vi "2_AdvancedDemo_MHHisto.vi"() -> ()   [LabVIEW 2017]
uses:
  Types/MH_InputChannel.ctl
  Types/MH_UIThread_Cmds.ctl
  Types/MH_UIThread_Data.ctl
  _lib/PQ/MultiHarp/MH_InitInfo.ctl
  _lib/PQ/MultiHarp/MH_RefSource.ctl
  _lib/PQ/MultiHarp/MH_MeasMode.ctl
  <vilib>/Utility/error.llb/DialogType.ctl
  _lib/PQ/MultiHarp/mhlib_x86_x64_UIThread.llb/MH_DllPath_global.vi
  <vilib>/Utility/error.llb/Error Cluster From Error Code.vi
  _lib/PQ/MultiHarp/MH_LibVersion_global.vi
  <vilib>/ErrorRing/Error Ring.xnode
panel:
  in  "Settings":bool=TRUE
  in  "Run continuously":bool=TRUE caption="Conti."
  in  "Start":bool
  in  "Scale":bool
  out "CountRates":i32[](graph)
  in  "HistoLength":i32(ring)=6 caption="Num Bins" items=["1024", "2048", "4096", "8192", "16384", "32768", "65536"]
  in  "OvlLevel":u32=100000 caption="Ovl.Level" min=1 step=1
  in  "StopOvl.":bool=TRUE
  in  "AcqTime":i32=1000 caption="Acqu.     ms" min=1 max=360000 step=1
  in  "Binning":i32(ring) caption="Resol.      ps" items=["80", "160", "320", "640", "1280", "2560", "5120", "10240", "20480", "40960", "81920", "163840", "327680", "655360", "1310720", "2621440", "5242880", "10485760", "20971520", "41943040", "83886080", "167772160", "335544320", "671088640", "1342177280", "2684354560"]
  in  "HistoOffset":i32 caption="Offset      ns" min=0 max=100000000 step=1
  out "HistoGraph":T1(graph)={0.0, "Resolution"=0.08, "Histogram"=[]}
  in  "SyncEdge":i32(ring) caption="Edge" items=["falling", "rising"]
  in  "SyncDivider":i32(ring)=3 caption="Divider" items=["1", "2", "4", "8", "16"]
  in  "SyncOffset":i32 caption="Offset      ps" min=-99999 max=99999 step=1
  in  "SyncLevel":i32=-50 caption="Level      mV" min=-1200 max=1200 step=1
  in  "Channels":T2[](array[typedef])=[{"Name"="Inp.Chan 1", "Enable"=TRUE, "Offset"=0, "Level"=-50, "Edge"=0}, {"Name"="Inp.Chan 2", "Enable"=TRUE, "Offset"=0, "Level"=-50, "Edge"=0}, {"Name"="Inp.Chan 3", "Enable"=TRUE, "Offset"=0, "Level"=-50, "Edge"=0}, {"Name"="Inp.Chan 4", "Enable"=TRUE, "Offset"=0, "Level"=-50, "Edge"=0}, {"Name"="Inp.Chan 5", "Enable"=TRUE, "Offset"=0, "Level"=-50, "Edge"=0}, {"Name"="Inp.Chan 6", "Enable"=TRUE, "Offset"=0, "Level"=-50, "Edge"=0}, {"Name"="Inp.Chan 7", "Enable"=TRUE, "Offset"=0, "Level"=-50, "Edge"=0}, {"Name"="Inp.Chan 8", "Enable"=TRUE, "Offset"=0, "Level"=-50, "Edge"=0}] {"Edge" items=["falling", "rising"]; "Offset" min=-99999 max=99999 step=80; "Level" min=-1200 max=1200 step=1}
  out "SyncRate":string="Sync Rate: 10000160 cps\n"
  out "OverFlow":bool caption="Overflow:"
  out "Status":string="Readout Rate: 7.4 Hz\t\tTotal Counts:\t\tCh. 1: 3766 cnts.\t\tCh. 2: 3766 cnts.\t\tCh. 3: 0 cnts.\t\tCh. 4: 0 cnts.\t\tCh. 5: 0 cnts.\t\tCh. 6: 0 cnts.\t\tCh. 7: 0 cnts.\t\tCh. 8: 0 cnts.\t\t"
  # "Histogram"
  # "Sync"
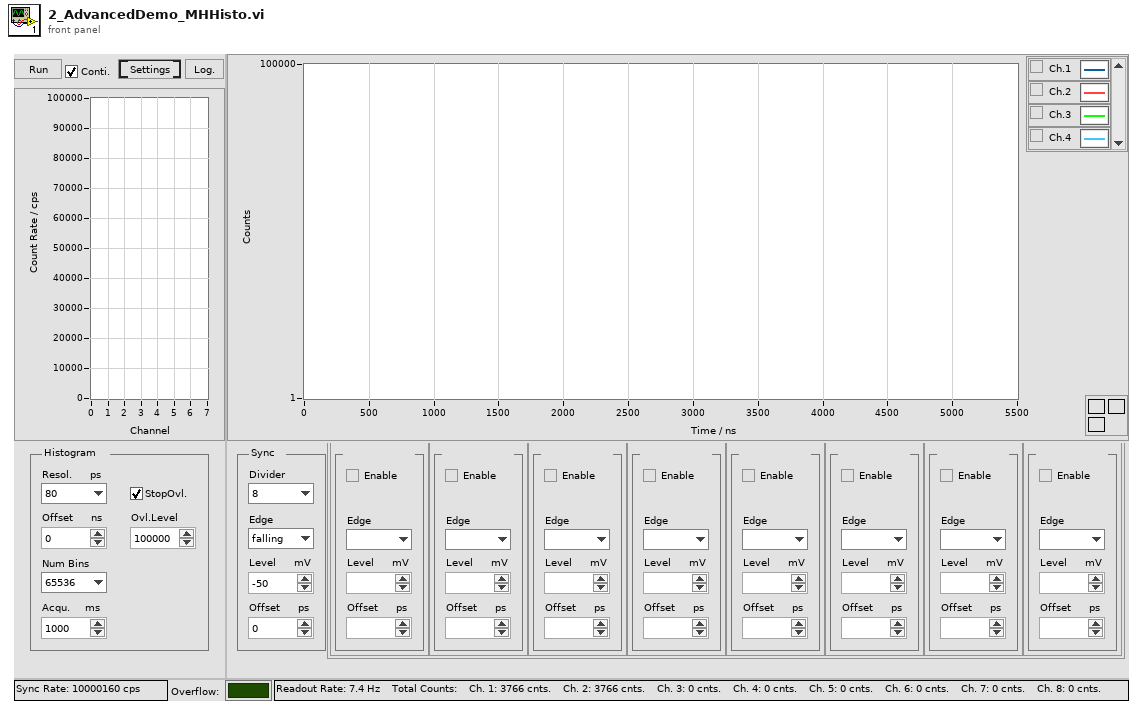
[diagram p1: front panel]
types:
  T1 = cluster{dbl, "Resolution":dbl, "Histogram":u32[][]}
  T2 = typedef "MH_InputChannel.ctl" = cluster{"Name":string, "Enable":bool, "Offset":i32, "Level":i32, "Edge":i32}
  T3 = typedef "MH_UIThread_Data.ctl" = cluster{"Init Info":T4, "DevIdx":i32, "SyncDivider":i32, "SyncOffset":i32, "SyncLevel":i32, "Channels":T2[], "CurrentChannels":i32[], "AcqTime":i32, "Binning":i32, "HistoOffset":i32, "HistoLen":i32, "StopOvl.":bool, "OvlLevel":u32, "SyncEdge":i32, "StartMeas":bool, "HistoLength":i32, "Resolution":dbl, "Run cont.":bool, "Status":string, "SyncRate":i32, "BitShift":i32, "HistoAcqTime":dbl}
  T4 = typedef "MH_InitInfo.ctl" = cluster{"Library Version":string, "Serial No.":string, "Model":string, "Partnum":string, "Version":string, "features":i32, "nchannels":i32, "Base Resolution":dbl, "Bin Steps":i32}
  T5 = typedef "MH_UIThread_Cmds.ctl" = enum16{"Idle", "Init", "SetInpChanEnable", "SetInpChanOffset", "SetInpChanTrg", "SetSyncDivider", "SetSyncTrg", "SetSyncOffset", "SetBinning", "SetHistoOffset", "SetHistoLen", "SetStopOvl", "SetBitShift", "SetHistoAcqTime", "GetRates", "GetAllRates", "StartMeas", "StopMeas", "AbortMeas", "GetResolution", "GetHistos", "GetAllHistos", "ReadFiFo", "WriteStatus", "Resize", "EnableControls", "DisableControls", "Error", "Exit"}
  T6 = enum8{"Enabled", "Disabled", "Disabled and Grayed Out"}
  T7 = typedef "MH_MeasMode.ctl" = i32
  T8 = typedef "MH_RefSource.ctl" = enum16{"INTERNAL", "EXTERNAL_10MHZ", "WR_MASTER_GENERIC", "WR_SLAVE_GENERIC", "WR_GRANDM_GENERIC", "EXTN_GPS_PPS", "EXTN_GPS_PPS_UART", "WR_MASTER_MHARP", "WR_SLAVE_MHARP", "WR_GRANDM_MHARP"}
  T9 = cluster{dbl, "Resolution":dbl, "Histograms":u32[][]}
  T10 = typedef "DialogType.ctl" = u16
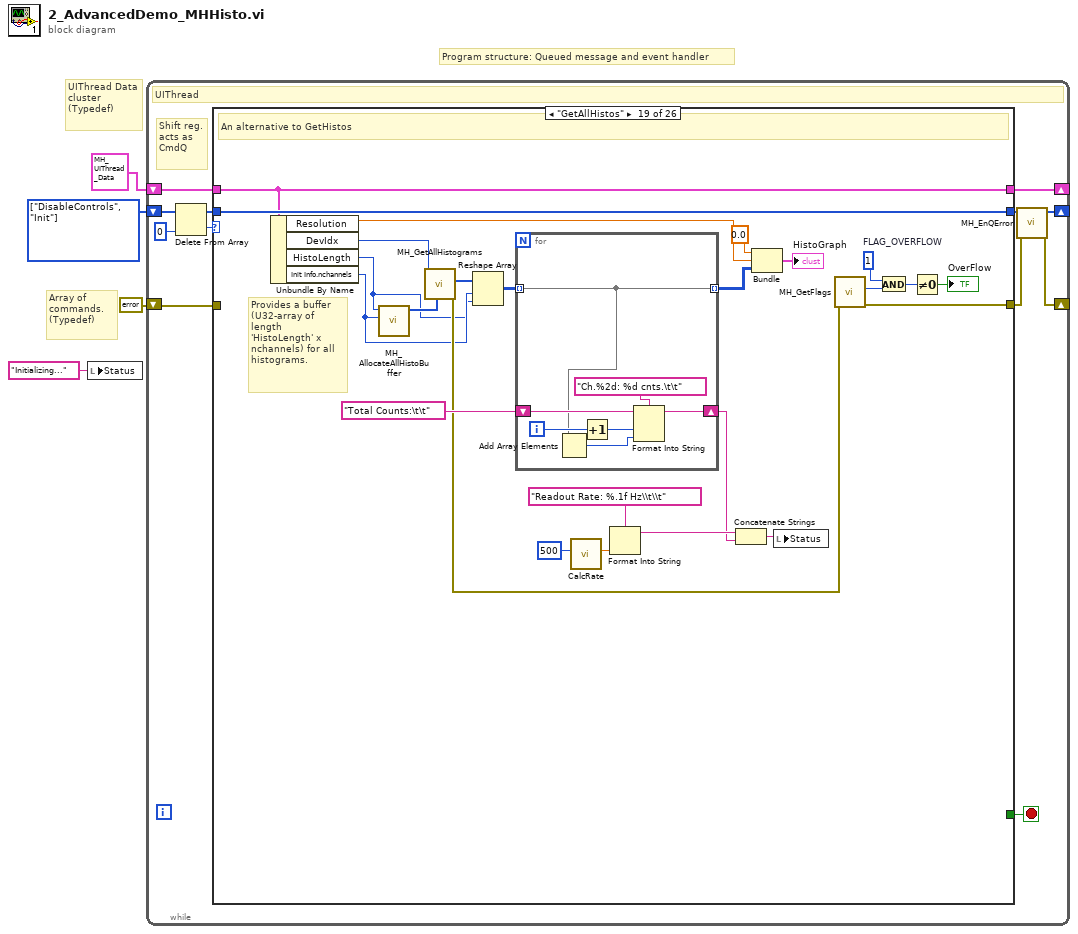
[diagram p0: block diagram]
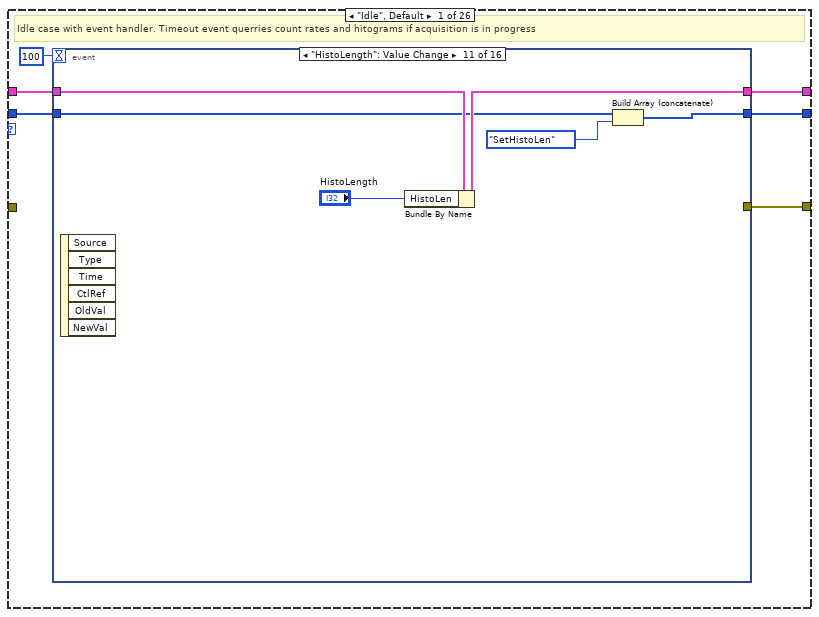
[diagram p2: hidden frame]
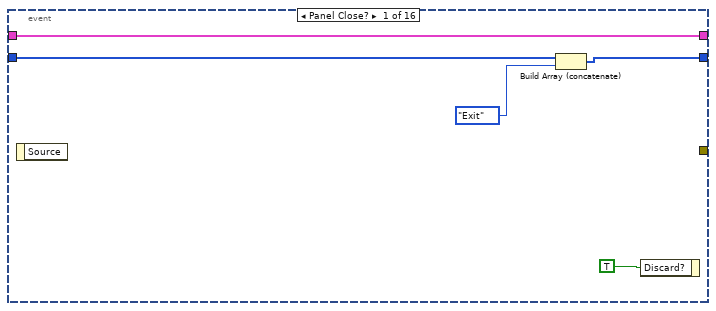
[diagram p3: hidden frame]
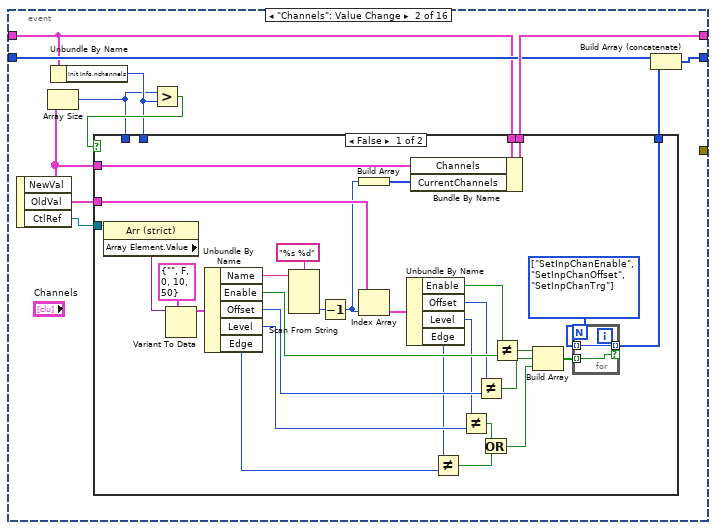
[diagram p4: hidden frame]
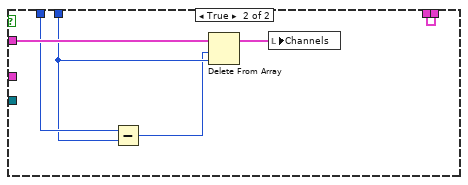
[diagram p5: hidden frame]
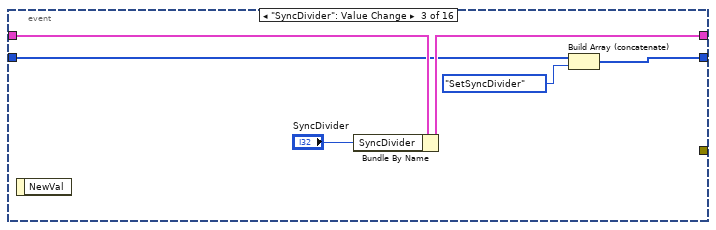
[diagram p6: hidden frame]
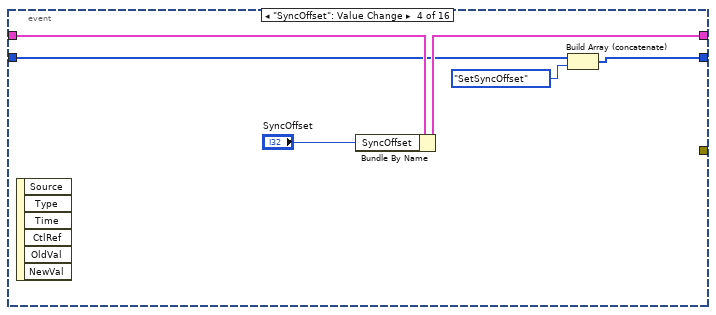
[diagram p7: hidden frame]
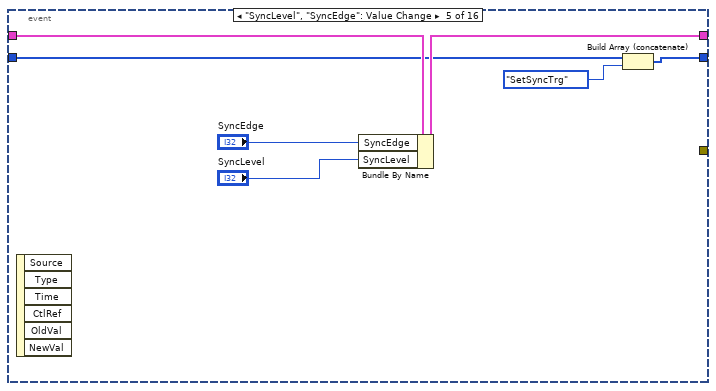
[diagram p8: hidden frame]
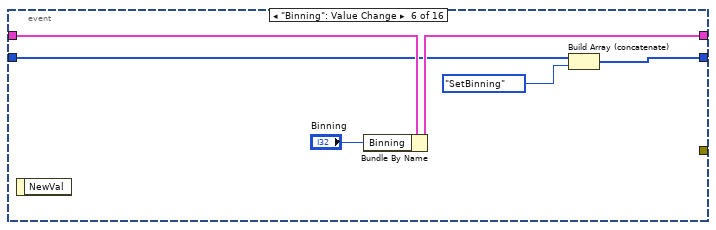
[diagram p9: hidden frame]
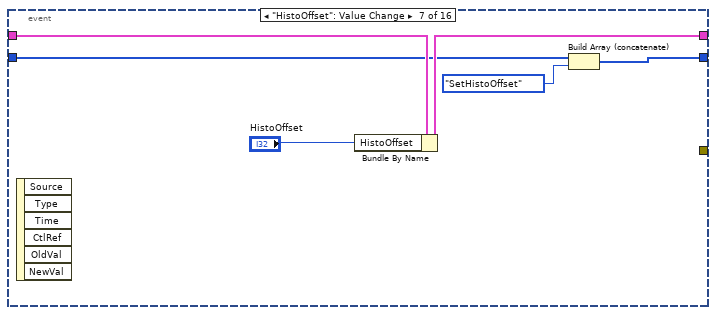
[diagram p10: hidden frame]
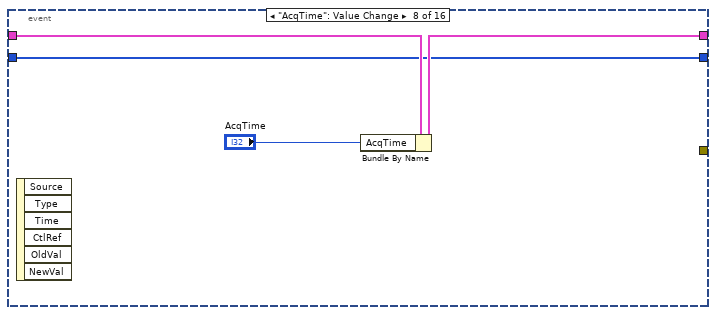
[diagram p11: hidden frame]
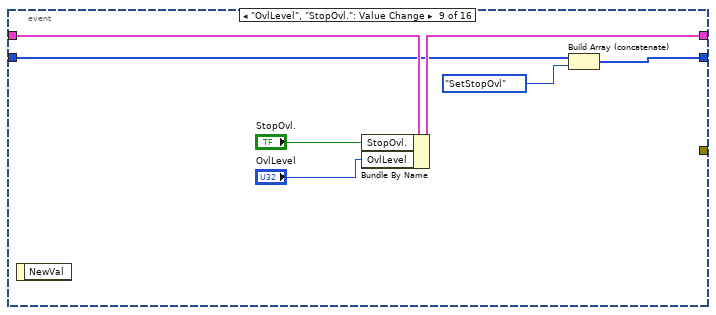
[diagram p12: hidden frame]
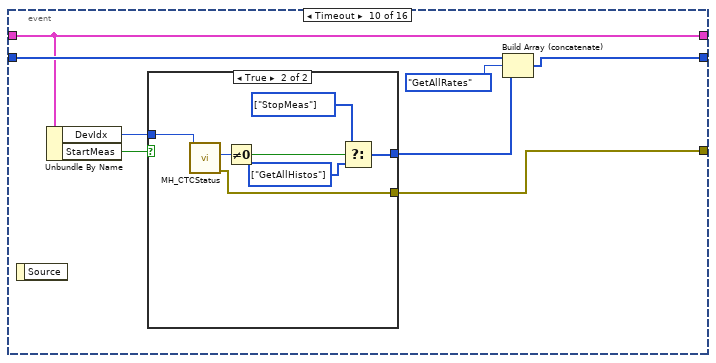
[diagram p13: hidden frame]
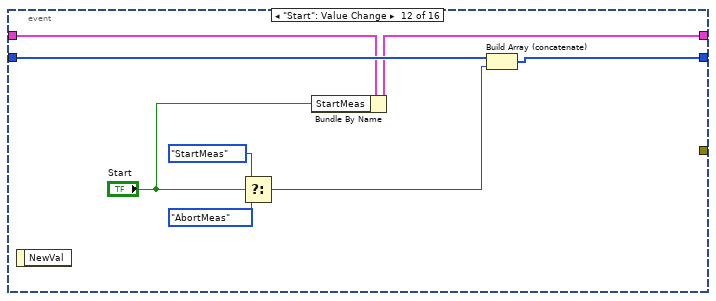
[diagram p15: hidden frame]
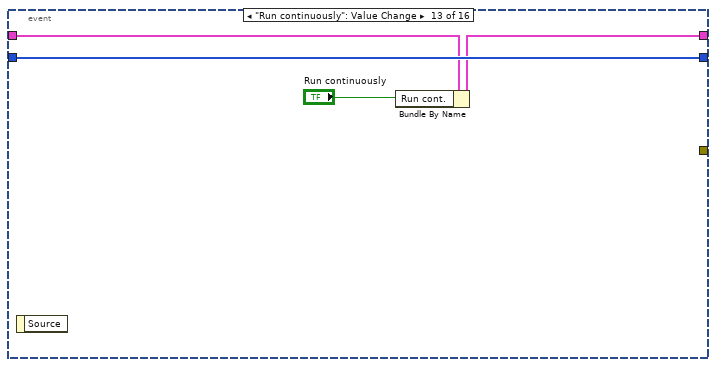
[diagram p16: hidden frame]
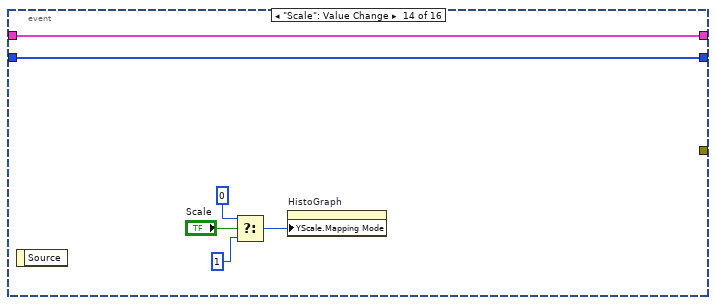
[diagram p17: hidden frame]
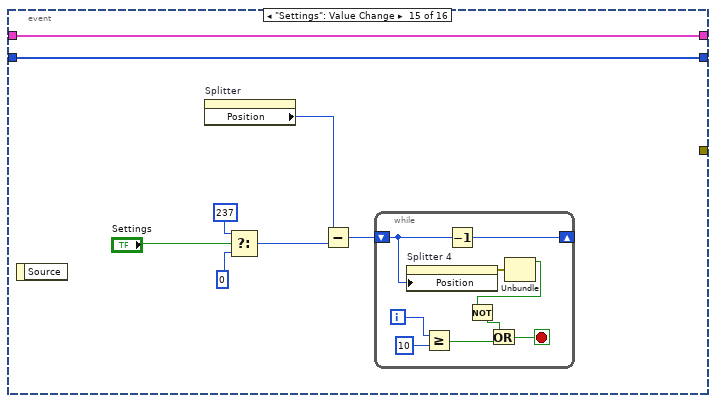
[diagram p18: hidden frame]
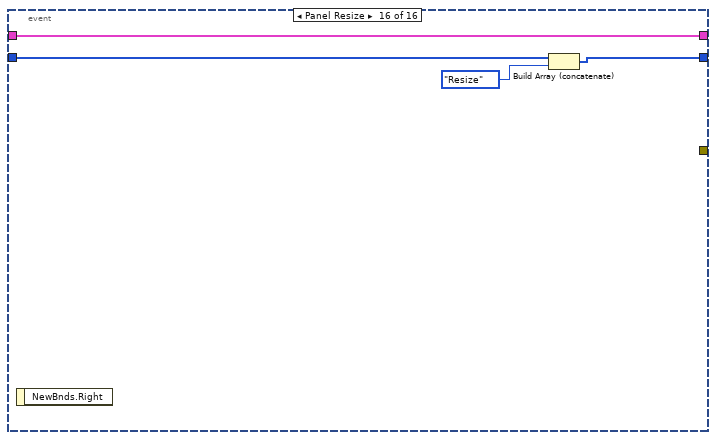
[diagram p19: hidden frame]
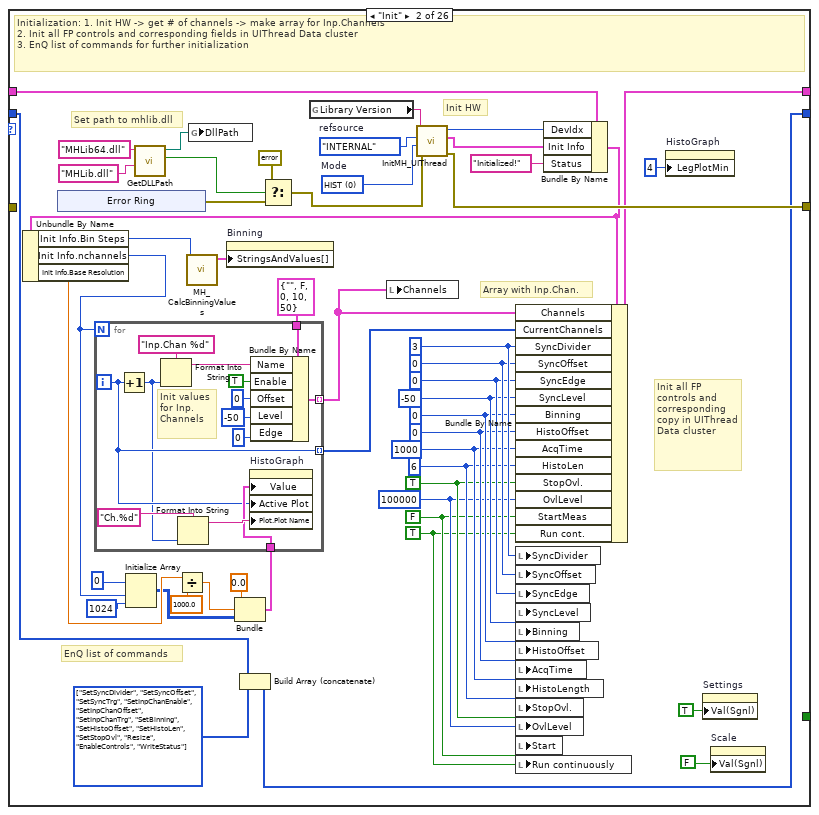
[diagram p20: hidden frame]
diagram:
  w3 = T5[] [enum."DisableControls", enum."Init"] items=["Idle", "Init", "SetInpChanEnable", "SetInpChanOffset", "SetInpChanTrg", "SetSyncDivider", "SetSyncTrg", "SetSyncOffset", "SetBinning", "SetHistoOffset", "SetHistoLen", "SetStopOvl", "SetBitShift", "SetHistoAcqTime", "GetRates", "GetAllRates", "StartMeas", "StopMeas", "AbortMeas", "GetResolution", "GetHistos", "GetAllHistos", "ReadFiFo", "WriteStatus", "Resize", "EnableControls", "DisableControls", "Error", "Exit"]
  # "Array of commands.\n(Typedef)"
  # "Program structure: Queued message and event handler"
  # "UIThread Data cluster\n(Typedef)"
  n1 = local write "Status"("Initializing..." ("Status")) -> ()
  n2 = while {
    shift-right: [w5] -> _
    shift-left: w3 -> [w12]
    shift-right: [w15] -> _
    shift-left: T3 {"Init Info"={"Library Version"="", "Serial No."="", "Model"="", "Partnum"="", "Version"="", "features"=0, "nchannels"=0, "Base Resolution"=0.0, "Bin Steps"=0}, "DevIdx"=0, "SyncDivider"=1, "SyncOffset"=0, "SyncLevel"=50, "Channels"=[], "CurrentChannels"=[], "AcqTime"=1, "Binning"=1, "HistoOffset"=1, "HistoLen"=1024, "StopOvl."=FALSE, "OvlLevel"=1024, "SyncEdge"=10, "StartMeas"=FALSE, "HistoLength"=0, "Resolution"=0.0, "Run cont."=FALSE, "Status"="", "SyncRate"=0, "BitShift"=0, "HistoAcqTime"=0.0} -> [w14]
    shift-right: [w7] -> _
    shift-left: errorcluster {"status"=FALSE, "code"=0, "source"=""} ("error IO") -> [w13]
    stop <- w16 stop-if-true
    # "Shift reg.\nacts as\nCmdQ"
    # "UIThread"
    n3 = Delete From Array(array=w12, index=0) -> (deleted portion=w10:T5, array with subset deleted=w9:T5[])  [unwired: 1 in]
    n4 = case shown="\"GetAllHistos\"" w10 {
      tunnel: [w22 w221 w249 w263 w277 w294 w303 w305 w312 w320 w328 w333 w344 w355 w370 w378 w392 w406 w431 w463 w487 w500 w507 w519 w525 w529] -> w6
      tunnel: [_ _ _ _ _ _ _ _ _ _ _ _ _ _ _ _ _ _ _ _ _ _ _ _ _ TRUE] -> w16
      tunnel: [w21 w201 w252 w266 w280 w296 w304 w309 w316 w321 w323 w334 w343 w354 w376 w381 w395 w402 w430 w462 w486 w488 w506 w518 w526 w532] -> w15
      tunnel: w14 -> [w20 w206 w252 w266 w280 w296 w304 w309 w316 w321 w324 w334 w343 w354 w376 w382 w396 w403 w430 w462 w486 w488 w506 w518 w526 w532]
      tunnel: [w17 w224 w250 w264 w278 w292 w302 w308 w315 w319 w327 w332 w337 w353 w375 w384 w398 w404 w428 w458 _ _ _ _ _ w530] -> w8
      tunnel: w13 -> [_ _ _ _ _ _ _ _ _ _ _ _ _ _ _ _ _ _ _ _ _ _ _ _ w527 _]
      tunnel: w9 -> [w19 w223 w249 w263 w277 w294 w303 w305 w311 w320 w328 w333 w344 w355 w371 w379 w393 w406 w431 w463 w487 w500 w507 w519 _ w529]
      frame "Idle", Default {
        # "Idle case with event handler. Timeout event querries count rates and hitograms if acquisition is in progress"
        n5 = event shown="[10] \"HistoLength\": Value Change" {
          selector: _ -> [_ _ _ _ _ _ _ _ _ _ _ _ _ _ _ _]
          dyn-events: _ -> [_ _ _ _ _ _ _ _ _ _ _ _ _ _ _ _]
          timeout: 100 -> [_ _ _ _ _ _ _ _ _ _ _ _ _ _ _ _]
          tunnel: [w23 w33 w77 w83 w90 w97 w103 w108 w114 w124 w135 w143 w151 w157 w165 w175] -> w22
          tunnel: [w26 w36 w81 w87 w94 w100 w106 w110 w117 w123 w138 w141 w149 w156 w164 w178] -> w21
          tunnel: w20 -> [w26 w32 w82 w88 w95 w101 w107 w111 w118 w123 w139 w142 w150 w156 w164 w178]
          tunnel: w19 -> [w25 w35 w79 w85 w92 w99 w105 w108 w116 w126 w137 w145 w151 w157 w165 w176]
          tunnel: [_ _ _ _ _ _ _ _ _ w119 _ _ _ _ _ _] -> w17
          event Panel Close? {
            n6 = event-data() -> ()  [unwired: 1 in, 1 out]
            n7 = Build Array (concatenate)(w25, MH_UIThread_Cmds."Exit") -> (w23:T5[])
            n8 = event-data("Discard?"=TRUE) -> ()  [unwired: 1 in, 1 out]
          }
          event "Channels": Value Change {
            n9 = event-data() -> ("NewVal"=w31:T2[], "OldVal"=w37:T2[], "CtlRef"=w38:refnum<vi>)  [unwired: 1 in]
            n10 = Array Size(array=w31) -> (size(s)=w28:i32)
            n11 = Unbundle By Name(w32) -> ("Init Info.nchannels"=w29:i32)
            n12 = Greater?(x=w28, y=w29) -> (0:w30:bool)
            n13 = case shown="False" w30 {
              tunnel: w38 -> [w68 _]
              tunnel: w37 -> [w62 _]
              tunnel: [w45 w76] -> w36
              tunnel: [w43 _] -> w34
              tunnel: w32 -> [w40 w76]
              tunnel: w31 -> [w39 w75]
              tunnel: w29 -> [_ w73]
              tunnel: w28 -> [_ w74]
              frame False {
                w46 = T5[] [enum."SetInpChanEnable", enum."SetInpChanOffset", enum."SetInpChanTrg"] items=["Idle", "Init", "SetInpChanEnable", "SetInpChanOffset", "SetInpChanTrg", "SetSyncDivider", "SetSyncTrg", "SetSyncOffset", "SetBinning", "SetHistoOffset", "SetHistoLen", "SetStopOvl", "SetBitShift", "SetHistoAcqTime", "GetRates", "GetAllRates", "StartMeas", "StopMeas", "AbortMeas", "GetResolution", "GetHistos", "GetAllHistos", "ReadFiFo", "WriteStatus", "Resize", "EnableControls", "DisableControls", "Error", "Exit"]
                n14 = property class="Arr (strict)"(reference=w68) -> ("Array Element.Value"=w67:variant)  [unwired: 1 in, 2 out]
                n15 = Variant To Data(type=T2 {"Name"="", "Enable"=FALSE, "Offset"=0, "Level"=10, "Edge"=50} ("Channel"), Variant=w67) -> (data=w44:T2)  [unwired: 1 in, 1 out]
                n16 = Unbundle By Name(w44) -> ("Name"=w65:string, "Enable"=w59:bool, "Offset"=w57:i32, "Level"=w55:i32, "Edge"=w53:i32)
                n17 = Scan From String(format string="%s %d", input string=w65) -> (output 2=w63:i32)  [unwired: 5 in, 3 out]
                n18 = Decrement(x=w63) -> (x-1=w42:i32)
                n19 = Build Array(w42) -> (w41:i32[])
                n20 = Index Array(array=w62, index=w42) -> (element=w61:T2)
                n21 = Unbundle By Name(w61) -> ("Enable"=w60:bool, "Offset"=w58:i32, "Level"=w56:i32, "Edge"=w54:i32)
                n22 = Bundle By Name(cluster=w40, "Channels"=w39, "CurrentChannels"=w41) -> (w45:T3)
                n23 = Not Equal?(x=w54, y=w53) -> (x != y?=w48:bool)
                n24 = Not Equal?(x=w56, y=w55) -> (x != y?=w49:bool)
                n25 = Not Equal?(x=w58, y=w57) -> (x != y?=w51:bool)
                n26 = Or(x=w49, y=w48) -> (x .or. y?=w47:bool)
                n27 = Not Equal?(x=w60, y=w59) -> (x != y?=w52:bool)
                n28 = Build Array(w52, w51, w47) -> (w50:bool[])
                n29 = for {
                  tunnel: w50 -> [w69] mode=indexing
                  tunnel: w46 -> [w70] mode=indexing
                  tunnel: [w70] -> w43 mode=indexing if=w69
                }
              }
              frame True {
                n30 = Subtract(x=w74, y=w73) -> (x-y=w72:i32)
                n31 = Delete From Array(array=w75, length=w72, index=w73) -> (array with subset deleted=w71:T2[])  [unwired: 1 out]
                n32 = local write "Channels"(w71) -> ()
              }
            }
            n33 = Build Array (concatenate)(w35, w34) -> (w33:T5[])
          }
          event "SyncDivider": Value Change {
            n34 = event-data() -> ()  [unwired: 1 in, 1 out]
            n35 = Bundle By Name(cluster=w82, "SyncDivider"="SyncDivider") -> (w81:T3)
            n36 = Build Array (concatenate)(w79, MH_UIThread_Cmds."SetSyncDivider") -> (w77:T5[])
          }
          event "SyncOffset": Value Change {
            n37 = event-data() -> ()  [unwired: 1 in, 6 out]
            n38 = Bundle By Name(cluster=w88, "SyncOffset"="SyncOffset") -> (w87:T3)
            n39 = Build Array (concatenate)(w85, MH_UIThread_Cmds."SetSyncOffset") -> (w83:T5[])
          }
          event "SyncLevel", "SyncEdge": Value Change {
            n40 = event-data() -> ()  [unwired: 1 in, 6 out]
            n41 = Bundle By Name(cluster=w95, "SyncEdge"="SyncEdge", "SyncLevel"="SyncLevel") -> (w94:T3)
            n42 = Build Array (concatenate)(w92, MH_UIThread_Cmds."SetSyncTrg") -> (w90:T5[])
          }
          event "Binning": Value Change {
            n43 = event-data() -> ()  [unwired: 1 in, 1 out]
            n44 = Bundle By Name(cluster=w101, "Binning"="Binning") -> (w100:T3)
            n45 = Build Array (concatenate)(w99, MH_UIThread_Cmds."SetBinning") -> (w97:T5[])
          }
          event "HistoOffset": Value Change {
            n46 = event-data() -> ()  [unwired: 1 in, 6 out]
            n47 = Bundle By Name(cluster=w107, "HistoOffset"="HistoOffset") -> (w106:T3)
            n48 = Build Array (concatenate)(w105, MH_UIThread_Cmds."SetHistoOffset") -> (w103:T5[])
          }
          event "AcqTime": Value Change {
            n49 = event-data() -> ()  [unwired: 1 in, 6 out]
            n50 = Bundle By Name(cluster=w111, "AcqTime"="AcqTime") -> (w110:T3)
          }
          event "OvlLevel", "StopOvl.": Value Change {
            n51 = event-data() -> ()  [unwired: 1 in, 1 out]
            n52 = Bundle By Name(cluster=w118, "StopOvl."="StopOvl.", "OvlLevel"="OvlLevel") -> (w117:T3)
            n53 = Build Array (concatenate)(w116, MH_UIThread_Cmds."SetStopOvl") -> (w114:T5[])
          }
          event Timeout {
            n54 = event-data() -> ()  [unwired: 1 in, 1 out]
            n55 = Unbundle By Name(w123) -> ("DevIdx"=w121:i32, "StartMeas"=w122:bool)
            n56 = case shown="True" w122 {
              tunnel: w121 -> [_ w133]
              tunnel: [_ w131] -> w120
              tunnel: [_ w128] -> w119
              frame False {
              }
              frame True {
                w129 = T5[] [enum."GetAllHistos"] items=["Idle", "Init", "SetInpChanEnable", "SetInpChanOffset", "SetInpChanTrg", "SetSyncDivider", "SetSyncTrg", "SetSyncOffset", "SetBinning", "SetHistoOffset", "SetHistoLen", "SetStopOvl", "SetBitShift", "SetHistoAcqTime", "GetRates", "GetAllRates", "StartMeas", "StopMeas", "AbortMeas", "GetResolution", "GetHistos", "GetAllHistos", "ReadFiFo", "WriteStatus", "Resize", "EnableControls", "DisableControls", "Error", "Exit"]
                w130 = T5[] [enum."StopMeas"] items=["Idle", "Init", "SetInpChanEnable", "SetInpChanOffset", "SetInpChanTrg", "SetSyncDivider", "SetSyncTrg", "SetSyncOffset", "SetBinning", "SetHistoOffset", "SetHistoLen", "SetStopOvl", "SetBitShift", "SetHistoAcqTime", "GetRates", "GetAllRates", "StartMeas", "StopMeas", "AbortMeas", "GetResolution", "GetHistos", "GetAllHistos", "ReadFiFo", "WriteStatus", "Resize", "EnableControls", "DisableControls", "Error", "Exit"]
                n57 = call "MH_CTCStatus.vi"("devidx"=w133) -> ("error out"=w128:errorcluster, "ctcstatus"=w132:i32)  [unwired: 8 in, 1 out]
                n58 = Not Equal To 0?(x=w132) -> (x != 0?=w127:bool)
                n59 = Select(t=w130, s=w127, f=w129) -> (s? t:f=w131:T5[])
              }
            }
            n60 = Build Array (concatenate)(w126, MH_UIThread_Cmds."GetAllRates", w120) -> (w124:T5[])
          }
          event "HistoLength": Value Change {
            n61 = event-data() -> ()  [unwired: 1 in, 6 out]
            n62 = Bundle By Name(cluster=w139, "HistoLen"="HistoLength") -> (w138:T3)
            n63 = Build Array (concatenate)(w137, MH_UIThread_Cmds."SetHistoLen") -> (w135:T5[])
          }
          event "Start": Value Change {
            n64 = event-data() -> ()  [unwired: 1 in, 1 out]
            n65 = Select(t=MH_UIThread_Cmds."StartMeas", s="Start", f=MH_UIThread_Cmds."AbortMeas") -> (s? t:f=w144:T5)
            n66 = Bundle By Name(cluster=w142, "StartMeas"="Start") -> (w141:T3)
            n67 = Build Array (concatenate)(w145, w144) -> (w143:T5[])
          }
          event "Run continuously": Value Change {
            n68 = event-data() -> ()  [unwired: 1 in, 1 out]
            n69 = Bundle By Name(cluster=w150, "Run cont."="Run continuously") -> (w149:T3)
          }
          event "Scale": Value Change {
            n70 = event-data() -> ()  [unwired: 1 in, 1 out]
            n71 = Select(t=u8 0 ("Y Scale.Mapping Mode"), s="Scale", f=u8 1 ("Y Scale.Mapping Mode")) -> (s? t:f=w152:u8)
            n72 = property on="HistoGraph" class="WFGraph (strict)"("YScale.Mapping Mode"=w152) -> ()  [unwired: 2 in, 2 out]
          }
          event "Settings": Value Change {
            n73 = event-data() -> ()  [unwired: 1 in, 1 out]
            n74 = property on="Splitter" class="Splitter"() -> ("Position"=w163:i32)  [unwired: 2 in, 2 out]
            n75 = Select(t=237 ("PosT"), s="Settings", f=0 ("PosF")) -> (s? t:f=w160:i32)
            n76 = Subtract(x=w163, y=w160) -> (x-y=w159:i32)
            n77 = while {
              shift-right: [w174] -> _
              shift-left: w159 -> [w167]
              i -> [w173]
              stop <- w170 stop-if-true
              n78 = property on="Splitter 4" class="Splitter"("Position"=w167) -> (error out=w166:errorcluster)  [unwired: 2 in, 1 out]
              n79 = Greater Or Equal?(x=w173, y=10) -> (x >= y?=w171:bool)
              n80 = Decrement(x=w167) -> (x-1=w174:i32)
              n81 = Unbundle(w166) -> ("status"=w169:bool)  [unwired: 2 out]
              n82 = Not(x=w169) -> (.not. x?=w168:bool)
              n83 = Or(x=w168, y=w171) -> (x .or. y?=w170:bool)
            }
          }
          event Panel Resize {
            n84 = event-data() -> ()  [unwired: 1 in, 1 out]
            n85 = Build Array (concatenate)(w176, MH_UIThread_Cmds."Resize") -> (w175:T5[])
          }
        }
      }
      frame "Init" {
        w179 = T7 0 items=["HIST"=0, "T2"=2, "T3"=3]  # Mode
        w193 = MH_RefSource."INTERNAL"  # refsource
        w208 = TRUE ("Run cont.")
        w210 = FALSE ("StartMeas")
        w211 = u32 100000 ("OvlLevel")
        w212 = TRUE ("StopOvl.")
        w213 = 6 ("HistoLen")
        w214 = 1000 ("AcqTime")
        w215 = 0 ("HistoOffset")
        w216 = 0 ("Binning")
        w217 = -50 ("SyncLevel")
        w218 = 0 ("SyncZeroX")
        w219 = 0 ("SyncOffset")
        w220 = 3 ("SyncDivider")
        w222 = T5[] [enum."SetSyncDivider", enum."SetSyncOffset", enum."SetSyncTrg", enum."SetInpChanEnable", enum."SetInpChanOffset", enum."SetInpChanTrg", enum."SetBinning", enum."SetHistoOffset", enum."SetHistoLen", enum."SetStopOvl", enum."Resize", enum."EnableControls", enum."WriteStatus"] items=["Idle", "Init", "SetInpChanEnable", "SetInpChanOffset", "SetInpChanTrg", "SetSyncDivider", "SetSyncTrg", "SetSyncOffset", "SetBinning", "SetHistoOffset", "SetHistoLen", "SetStopOvl", "SetBitShift", "SetHistoAcqTime", "GetRates", "GetAllRates", "StartMeas", "StopMeas", "AbortMeas", "GetResolution", "GetHistos", "GetAllHistos", "ReadFiFo", "WriteStatus", "Resize", "EnableControls", "DisableControls", "Error", "Exit"]
        # "Init HW"
        # "Set path to mhlib.dll"
        # "Init all FP controls and corresponding copy in UIThread Data cluster"
        # "EnQ list of commands"
        # "Array with Inp.Chan."
        # "Initialization: 1. Init HW -> get # of channels -> make array for Inp.Channels\n2. Init all FP controls and corresponding fields in UIThread Data cluster\n3. EnQ list of commands for further initialization"
        n86 = xnode "Error Ring"() -> ("error out"=w194:errorcluster)
        n87 = call "GetDLLPath.vi"("DllName_32bit"="MHLib.dll" ("name or relative path"), "DllName_64bit"="MHLib64.dll" ("name or relative path")) -> ("file exists?"=w196:bool, "DLLPath"=w197:path)  [unwired: 8 in]
        n88 = global write "MH_DllPath_global.vi" "DllPath"(w197) -> ()
        n89 = Build Array (concatenate)(w223, w222) -> (w221:T5[])
        n90 = Select(t=errorcluster {"status"=FALSE, "code"=0, "source"=""} ("error IO"), s=w196, f=w194) -> (s? t:f=w202:errorcluster)
        n91 = global read "MH_LibVersion_global.vi" "Library Version"() -> (w192:string)
        n92 = call "InitMH_UIThread.vi"("error in (no error)"=w202, "Mode"=w179, "refsource"=w193, "Library Version"=w192) -> ("error out"=w224:errorcluster, "Init Info"=w227:T4, "DevIdx"=w226:i32)  [unwired: 5 in]
        n93 = local write "SyncDivider"(w220) -> ()
        n94 = local write "SyncOffset"(w219) -> ()
        n95 = local write "SyncEdge"(w218) -> ()
        n96 = local write "SyncLevel"(w217) -> ()
        n97 = local write "Binning"(w216) -> ()
        n98 = local write "HistoOffset"(w215) -> ()
        n99 = local write "AcqTime"(w214) -> ()
        n100 = local write "HistoLength"(w213) -> ()
        n101 = local write "StopOvl."(w212) -> ()
        n102 = local write "OvlLevel"(w211) -> ()
        n103 = local write "Start"(w210) -> ()
        n104 = local write "Run continuously"(w208) -> ()
        n105 = Bundle By Name(cluster=w206, "DevIdx"=w226, "Init Info"=w227, "Status"="Initialized!") -> (w205:T3)
        n106 = Unbundle By Name(w205) -> ("Init Info.Bin Steps"=w204:i32, "Init Info.nchannels"=w181:i32, "Init Info.Base Resolution"=w186:dbl)
        n107 = Initialize Array(u32 0, w181, 1024 ("dimension size")) -> (w185:u32[][])
        n108 = Divide(x=w186, y=1000.0) -> (x/y=w187:dbl)
        n109 = call "MH_CalcBinningValues.vi"("Bin Steps"=w204) -> ("BinningValues"=w209:cluster{"String":string, "Value":i32}[])  [unwired: 10 in]
        n110 = property on="Binning" class="Ring (strict)"("StringsAndValues[]"=w209) -> ()  [unwired: 2 in, 2 out]
        n111 = Bundle(0.0, w187, w185) -> (w184:cluster{dbl, dbl, u32[][]})  [unwired: 1 in]
        n112 = for {
          N: w181 -> [_]
          tunnel: T2 {"Name"="", "Enable"=FALSE, "Offset"=0, "Level"=10, "Edge"=50} ("Channel") -> [w245]
          tunnel: [w244] -> w180 mode=indexing
          tunnel: [w234] -> w182 mode=indexing
          tunnel: w184 -> [w235]
          i -> [w234]
          # "Init values for Inp. Channels"
          n113 = Increment(x=w234) -> (x+1=w233:i32)
          n114 = Format Into String(format string="Inp.Chan %d", w233) -> (resulting string=w242:string)  [unwired: 2 in, 1 out]
          n115 = Format Into String(format string="Ch.%d", w233) -> (resulting string=w236:string)  [unwired: 2 in, 1 out]
          n116 = property on="HistoGraph" class="WFGraph (strict)"("Value"=w235, "Active Plot"=w234, "Plot.Plot Name"=w236) -> ()  [unwired: 2 in, 2 out]
          n117 = Bundle By Name(cluster=w245, "Name"=w242, "Enable"=TRUE, "Offset"=0, "Level"=-50 ("CFDZeroX"), "Edge"=0 ("CFDLevel")) -> (w244:T2)
        }
        n118 = local write "Channels"(w180) -> ()
        n119 = Bundle By Name(cluster=w205, "Channels"=w180, "CurrentChannels"=w182, "SyncDivider"=w220, "SyncOffset"=w219, "SyncEdge"=w218, "SyncLevel"=w217, "Binning"=w216, "HistoOffset"=w215, "AcqTime"=w214, "HistoLen"=w213, "StopOvl."=w212, "OvlLevel"=w211, "StartMeas"=w210, "Run cont."=w208) -> (w201:T3)
        n120 = property on="HistoGraph" class="WFGraph (strict)"("LegPlotMin"=u32 4 ("Legend:Plot Minimum")) -> ()  [unwired: 2 in, 2 out]
        n121 = property on="Settings" class="Bool (strict)"("Val(Sgnl)"=TRUE ("Value (Signaling)")) -> ()  [unwired: 2 in, 2 out]
        n122 = property on="Scale" class="Bool (strict)"("Val(Sgnl)"=FALSE ("Value (Signaling)")) -> ()  [unwired: 2 in, 2 out]
      }
      frame "SetInpChanEnable" {
        n123 = Unbundle By Name(w252) -> ("DevIdx"=w251:i32, "Channels"=w246:T2[], "CurrentChannels"=w247:i32[])
        n124 = for {
          tunnel: w251 -> [w259]
          shift-right: [w258] -> w250
          shift-left: errorcluster {"status"=FALSE, "code"=0, "source"=""} ("error out") -> [w257]
          tunnel: w247 -> [w253] mode=indexing
          tunnel: w246 -> [w256]
          n125 = Index Array(array=w256, index=w253) -> (element=w255:T2)
          n126 = Unbundle By Name(w255) -> ("Enable"=w254:bool)
          n127 = call "MH_SetInputChannelEnable.vi"("error in (no error)"=w257, "enable"=w254, "channel"=w253, "devidx"=w259) -> ("error out"=w258:errorcluster)  [unwired: 6 in, 1 out]
        }
      }
      frame "SetInpChanOffset" {
        n128 = Unbundle By Name(w266) -> ("DevIdx"=w265:i32, "Channels"=w260:T2[], "CurrentChannels"=w261:i32[])
        n129 = for {
          tunnel: w265 -> [w271]
          shift-right: [w268] -> w264
          shift-left: errorcluster {"status"=FALSE, "code"=0, "source"=""} ("error out") -> [w269]
          tunnel: w261 -> [w270] mode=indexing
          tunnel: w260 -> [w273]
          n130 = Index Array(array=w273, index=w270) -> (element=w272:T2)
          n131 = Unbundle By Name(w272) -> ("Offset"=w267:i32)
          n132 = call "MH_SetInputChannelOffset.vi"("error in (no error)"=w269, "Offset"=w267, "channel"=w270, "devidx"=w271) -> ("error out"=w268:errorcluster)  [unwired: 6 in, 1 out]
        }
      }
      frame "SetInpChanTrg" {
        n133 = Unbundle By Name(w280) -> ("DevIdx"=w279:i32, "Channels"=w274:T2[], "CurrentChannels"=w275:i32[])
        n134 = for {
          tunnel: w279 -> [w283]
          shift-right: [w285] -> w278
          shift-left: errorcluster {"status"=FALSE, "code"=0, "source"=""} ("error out") -> [w286]
          tunnel: w275 -> [w284] mode=indexing
          tunnel: w274 -> [w288]
          n135 = Index Array(array=w288, index=w284) -> (element=w287:T2)
          n136 = Unbundle By Name(w287) -> ("Level"=w282:i32, "Edge"=w281:i32)
          n137 = call "MH_SetInputEdgeTrg.vi"("channel"=w284, "error in (no error)"=w286, "edge"=w281, "level"=w282, "devidx"=w283) -> ("error out"=w285:errorcluster)  [unwired: 5 in, 1 out]
        }
      }
      frame "SetSyncDivider" {
        n138 = Unbundle By Name(w296) -> ("DevIdx"=w295:i32, "SyncDivider"=w291:i32)
        n139 = Power Of 2(x=w291) -> (2^x=w290:dbl)
        n140 = To Long Integer(number=w290) -> (32bit integer=w289:i32)
        n141 = call "MH_SetSyncDiv.vi"("SyncDivider"=w289, "devidx"=w295) -> ("error out"=w293:errorcluster)  [unwired: 8 in, 1 out]
        n142 = flat-sequence {
          tunnel: w293 -> [w297]
          tunnel: [w297] -> w292
          frame #0 {
            n143 = Wait (ms)(milliseconds to wait=u32 100) -> ()  [unwired: 1 out]
          }
        }
      }
      frame "SetSyncTrg" {
        n144 = Unbundle By Name(w304) -> ("DevIdx"=w301:i32, "SyncLevel"=w299:i32, "SyncEdge"=w300:i32)
        n145 = call "MH_SetSyncEdgeTrg.vi"("edge"=w300, "level"=w299, "devidx"=w301) -> ("error out"=w302:errorcluster)  [unwired: 7 in, 1 out]
      }
      frame "SetSyncOffset" {
        n146 = Unbundle By Name(w309) -> ("DevIdx"=w307:i32, "SyncOffset"=w306:i32)
        n147 = call "MH_SetSyncChannelOffset.vi"("Offset"=w306, "devidx"=w307) -> ("error out"=w308:errorcluster)  [unwired: 8 in, 1 out]
      }
      frame "SetBinning" {
        # "When binning is changed the new resolution is querried"
        n148 = Unbundle By Name(w316) -> ("DevIdx"=w314:i32, "Binning"=w313:i32)
        n149 = call "MH_SetBinning.vi"("Binning"=w313, "devidx"=w314) -> ("error out"=w315:errorcluster)  [unwired: 8 in, 1 out]
        n150 = Build Array (concatenate)(MH_UIThread_Cmds."GetResolution", w311) -> (w312:T5[])
      }
      frame "SetHistoOffset" {
        n151 = Unbundle By Name(w321) -> ("DevIdx"=w318:i32, "HistoOffset"=w317:i32)
        n152 = call "MH_SetOffset.vi"("Offset"=w317, "devidx"=w318) -> ("error out"=w319:errorcluster)  [unwired: 8 in, 1 out]
      }
      frame "SetHistoLen" {
        n153 = Unbundle By Name(w324) -> ("DevIdx"=w326:i32, "HistoLen"=w325:i32)
        n154 = call "MH_SetHistoLen.vi"("lencode"=w325, "devidx"=w326) -> ("error out"=w327:errorcluster, "actuallen"=w322:i32)  [unwired: 7 in, 1 out]
        n155 = Bundle By Name(cluster=w324, "HistoLength"=w322) -> (w323:T3)
      }
      frame "SetStopOvl" {
        n156 = Unbundle By Name(w334) -> ("DevIdx"=w331:i32, "StopOvl."=w330:bool, "OvlLevel"=w329:u32)
        n157 = call "MH_SetStopOverflow.vi"("stopcount"=w329, "StopOnOverflow"=w330, "devidx"=w331) -> ("error out"=w332:errorcluster)  [unwired: 7 in, 1 out]
      }
      frame "GetAllRates" {
        # "An alternative to GetRates"
        n158 = Unbundle By Name(w343) -> ("DevIdx"=w340:i32, "Init Info.nchannels"=w335:i32)
        n159 = call "MH_AllocateCntRateBuffer.vi"("NumChan"=w335) -> ("Buffer"=w336:i32[])  [unwired: 10 in]
        n160 = call "MH_GetAllCountRates.vi"("cntrates_buf"=w336, "devidx"=w340) -> ("error out"=w337:errorcluster, "cntrates"=→"CountRates":i32[], "syncrate"=w339:i32)  [unwired: 6 in, 1 out]
        n161 = Format Into String(format string="Sync Rate: %d cps\n", w339) -> (resulting string=→"SyncRate":string)  [unwired: 2 in, 1 out]
      }
      frame "GetRates" {
        # "An alternative to GetAllRates"
        n162 = Unbundle By Name(w354) -> ("Init Info.nchannels"=w349:i32, "Channels"=w351:T2[], "DevIdx"=w350:i32)
        n163 = call "MH_GetSyncRate.vi"("devidx"=w350) -> ("error out"=w347:errorcluster, "syncrate"=w346:i32)  [unwired: 8 in, 1 out]
        n164 = Format Into String(format string="Sync Rate: %d cps\n", w346) -> (resulting string=w348:string)  [unwired: 2 in, 1 out]
        n165 = for {
          N: w349 -> [_]
          tunnel: w350 -> [w361]
          tunnel: [w358] -> w345 mode=indexing
          shift-right: [w360] -> w353
          shift-left: w347 -> [w362]
          tunnel: w351 -> [w357] mode=indexing
          i -> [w359]
          n166 = Unbundle By Name(w357) -> ("Enable"=w356:bool)
          n167 = case shown="True" w356 {
            tunnel: w362 -> [w363 w368]
            tunnel: w361 -> [_ w367]
            tunnel: [w363 w366] -> w360
            tunnel: w359 -> [_ w365]
            tunnel: [_ w364] -> w358
            frame False {
            }
            frame True {
              n168 = call "MH_GetCountRate.vi"("error in (no error)"=w368, "Channel"=w365, "devidx"=w367) -> ("error out"=w366:errorcluster, "rate"=w364:i32)  [unwired: 6 in, 1 out]
            }
          }
        }
        n169 = local write "SyncRate"(w348) -> ()
        n170 = local write "CountRates"(w345) -> ()
      }
      frame "StartMeas" {
        n171 = Unbundle By Name(w376) -> ("AcqTime"=w372:i32, "DevIdx"=w373:i32)
        n172 = call "MH_ClearHistMem.vi"("devidx"=w373) -> ("error out"=w374:errorcluster)  [unwired: 9 in, 1 out]
        n173 = call "MH_StartMeas.vi"("error in (no error)"=w374, "tacq"=w372, "devidx"=w373) -> ("error out"=w375:errorcluster)  [unwired: 7 in, 1 out]
        n174 = Build Array (concatenate)(w371, MH_UIThread_Cmds."GetAllHistos") -> (w370:T5[])
      }
      frame "StopMeas" {
        n175 = Unbundle By Name(w382) -> ("Run cont."=w377:bool, "DevIdx"=w383:i32)
        n176 = call "MH_StopMeas.vi"("devidx"=w383) -> ("error out"=w384:errorcluster)  [unwired: 9 in, 1 out]
        n177 = case shown="True" w377 {
          tunnel: w382 -> [w388 w390]
          tunnel: [w387 w390] -> w381
          tunnel: [w385 w389] -> w380
          frame False {
            w385 = T5[] [enum."GetAllHistos"] items=["Idle", "Init", "SetInpChanEnable", "SetInpChanOffset", "SetInpChanTrg", "SetSyncDivider", "SetSyncTrg", "SetSyncOffset", "SetBinning", "SetHistoOffset", "SetHistoLen", "SetStopOvl", "SetBitShift", "SetHistoAcqTime", "GetRates", "GetAllRates", "StartMeas", "StopMeas", "AbortMeas", "GetResolution", "GetHistos", "GetAllHistos", "ReadFiFo", "WriteStatus", "Resize", "EnableControls", "DisableControls", "Error", "Exit"]
            w386 = FALSE ("StartMeas")
            n178 = Bundle By Name(cluster=w388, "StartMeas"=w386) -> (w387:T3)
            n179 = local write "Start"(w386) -> ()
          }
          frame True {
            w389 = T5[] [enum."GetAllHistos", enum."StartMeas"] items=["Idle", "Init", "SetInpChanEnable", "SetInpChanOffset", "SetInpChanTrg", "SetSyncDivider", "SetSyncTrg", "SetSyncOffset", "SetBinning", "SetHistoOffset", "SetHistoLen", "SetStopOvl", "SetBitShift", "SetHistoAcqTime", "GetRates", "GetAllRates", "StartMeas", "StopMeas", "AbortMeas", "GetResolution", "GetHistos", "GetAllHistos", "ReadFiFo", "WriteStatus", "Resize", "EnableControls", "DisableControls", "Error", "Exit"]
          }
        }
        n180 = Build Array (concatenate)(w379, w380) -> (w378:T5[])
      }
      frame "AbortMeas" {
        w394 = T5[] [enum."GetAllHistos"] items=["Idle", "Init", "SetInpChanEnable", "SetInpChanOffset", "SetInpChanTrg", "SetSyncDivider", "SetSyncTrg", "SetSyncOffset", "SetBinning", "SetHistoOffset", "SetHistoLen", "SetStopOvl", "SetBitShift", "SetHistoAcqTime", "GetRates", "GetAllRates", "StartMeas", "StopMeas", "AbortMeas", "GetResolution", "GetHistos", "GetAllHistos", "ReadFiFo", "WriteStatus", "Resize", "EnableControls", "DisableControls", "Error", "Exit"]
        w391 = FALSE ("StartMeas")
        n181 = Unbundle By Name(w396) -> ("DevIdx"=w397:i32)
        n182 = call "MH_StopMeas.vi"("devidx"=w397) -> ("error out"=w398:errorcluster)  [unwired: 9 in, 1 out]
        n183 = Bundle By Name(cluster=w396, "StartMeas"=w391) -> (w395:T3)
        n184 = local write "Start"(w391) -> ()
        n185 = Build Array (concatenate)(w393, w394) -> (w392:T5[])
      }
      frame "GetResolution" {
        # "Resolution in ns"
        # "Gets resolution in ps"
        # "Resolution is saved in UIThread Data cluster in ns"
        n186 = Unbundle By Name(w403) -> ("DevIdx"=w405:i32)
        n187 = call "MH_GetResolution.vi"("devidx"=w405) -> ("error out"=w404:errorcluster, "resolution"=w401:dbl)  [unwired: 8 in, 1 out]
        n188 = Divide(x=w401, y=1000.0) -> (x/y=w399:dbl)
        n189 = Bundle By Name(cluster=w403, "Resolution"=w399) -> (w402:T3)
      }
      frame "GetAllHistos" {
        w419 = 1  # FLAG_OVERFLOW
        # "Provides a buffer (U32-array of length 'HistoLength' x nchannels) for all histograms."
        # "An alternative to GetHistos"
        n190 = Unbundle By Name(w430) -> ("Resolution"=w429:dbl, "DevIdx"=w411:i32, "HistoLength"=w407:i32, "Init Info.nchannels"=w408:i32)
        n191 = call "MH_AllocateAllHistoBuffer.vi"("NumChan"=w408, "HistoLength"=w407) -> ("Buffer"=w410:u32[])  [unwired: 9 in]
        n192 = call "MH_GetAllHistograms.vi"("Chcount"=w410, "devidx"=w411) -> ("error out"=w409:errorcluster, "Histograms"=w413:u32[])  [unwired: 7 in, 1 out]
        n193 = Reshape Array(w413, w408, w407) -> (w412:u32[][])
        n194 = for {
          tunnel: [w432] -> w421 mode=indexing
          shift-right: [w434] -> w415
          shift-left: "Total Counts:\t\t" -> [w433]
          tunnel: w412 -> [w432] mode=indexing
          i -> [w438]
          n195 = Add Array Elements(numeric array=w432) -> (sum=w435:u32)
          n196 = Increment(x=w438) -> (x+1=w436:i32)
          n197 = Format Into String(format string="Ch.%2d: %d cnts.\t\t", initial string=w433, w436, w435) -> (resulting string=w434:string)  [unwired: 1 in, 1 out]
        }
        n198 = call "CalcRate.vi"("Refresh(ms)"=u32 500) -> ("Rate / Hz"=w427:dbl)  [unwired: 8 in, 2 out]
        n199 = Format Into String(format string="Readout Rate: %.1f Hz\\t\\t", w427) -> (resulting string=w425:string)  [unwired: 2 in, 1 out]
        n200 = Concatenate Strings(w425, w415) -> (w424:string)
        n201 = Bundle(0.0, "Resolution"=w429, "Histograms"=w421) -> (→"HistoGraph":T9)  [unwired: 1 in]
        n202 = local write "Status"(w424) -> ()
        n203 = call "MH_GetFlags.vi"("error in (no error)"=w409) -> ("error out"=w428:errorcluster, "flags"=w418:i32)  [unwired: 8 in, 1 out]
        n204 = And(x=w419, y=w418) -> (x .and. y?=w420:i32)
        n205 = Not Equal To 0?(x=w420) -> (x != 0?=→"OverFlow":bool)
      }
      frame "GetHistos" {
        w448 = 1  # FLAG_OVERFLOW
        # "Provides a buffer (U32-array of length 'HistoLength') for histograms."
        # "An alternative to GetAllHistos"
        n206 = Unbundle By Name(w462) -> ("Resolution"=w459:dbl, "Init Info.nchannels"=w441:i32, "Channels"=w442:T2[], "DevIdx"=w461:i32, "HistoLength"=w460:i32)
        n207 = call "MH_AllocateHistoBuffer.vi"("HistoLength"=w460) -> ("Buffer"=w453:u32[])  [unwired: 10 in]
        n208 = for {
          N: w441 -> [_]
          tunnel: w461 -> [w476]
          tunnel: [w473] -> w451 mode=indexing
          tunnel: w453 -> [w474]
          shift-right: [w475] -> w450
          shift-left: errorcluster {"status"=FALSE, "code"=0, "source"=""} ("error IO") -> [w467]
          shift-right: [w468] -> w444
          shift-left: "Total Counts:\t\t" -> [w466]
          tunnel: w442 -> [w465] mode=indexing
          i -> [w472]
          n209 = Unbundle By Name(w465) -> ("Enable"=w464:bool)
          n210 = case shown="True" w464 {
            tunnel: w476 -> [_ w484]
            tunnel: [w477 w483] -> w475
            tunnel: w474 -> [w478 w482]
            tunnel: [w478 w481] -> w473
            tunnel: w472 -> [_ w480]
            tunnel: w467 -> [w477 w479]
            frame False {
            }
            frame True {
              n211 = call "MH_GetHistogram.vi"("Chcount"=w482, "error in (no error)"=w479, "channel"=w480, "devidx"=w484) -> ("error out"=w483:errorcluster, "Histogram"=w481:u32[])  [unwired: 5 in, 1 out]
            }
          }
          n212 = Add Array Elements(numeric array=w473) -> (sum=w469:u32)
          n213 = Increment(x=w472) -> (x+1=w470:i32)
          n214 = Format Into String(format string="Ch.%2d: %d cnts.\t\t", initial string=w466, w470, w469) -> (resulting string=w468:string)  [unwired: 1 in, 1 out]
        }
        n215 = call "CalcRate.vi"("Refresh(ms)"=u32 500) -> ("Rate / Hz"=w457:dbl)  [unwired: 8 in, 2 out]
        n216 = Format Into String(format string="Readout Rate: %.1f Hz\\t\\t", w457) -> (resulting string=w455:string)  [unwired: 2 in, 1 out]
        n217 = Concatenate Strings(w455, w444) -> (w454:string)
        n218 = Bundle(0.0, "Resolution"=w459, "Histogram"=w451) -> (w439:T1)  [unwired: 1 in]
        n219 = local write "HistoGraph"(w439) -> ()
        n220 = local write "Status"(w454) -> ()
        n221 = call "MH_GetFlags.vi"("error in (no error)"=w450) -> ("error out"=w458:errorcluster, "flags"=w447:i32)  [unwired: 8 in, 1 out]
        n222 = And(x=w448, y=w447) -> (x .and. y?=w449:i32)
        n223 = Not Equal To 0?(x=w449) -> (x != 0?=w440:bool)
        n224 = local write "OverFlow"(w440) -> ()
      }
      frame "WriteStatus" {
        n225 = Unbundle By Name(w486) -> ("Status"=→"Status":string)
      }
      frame "Resize" {
        n226 = property on="Pane 3" class="Pane"() -> ("Width"=w493:u32)  [unwired: 2 in, 2 out]
        n227 = Subtract(x=w493, y=i16 100 ("b")) -> (x-y=w499:u32)
        n228 = Unbundle By Name(w488) -> ("Init Info.nchannels"=w496:i32)
        n229 = Quotient & Remainder(x=w499, y=i16 99 ("m")) -> (floor(x/y)=w498:u32)  [unwired: 1 out]
        n230 = In Range and Coerce(upper limit=w496, x=w498, lower limit=4) -> (coerced(x)=w497:u32)  [unwired: 1 out]
        n231 = Equal?(x=w496, y=w497) -> (x = y?=w495:bool)
        n232 = Not(x=w495) -> (.not. x?=w494:bool)
        n233 = property on="Channels" class="Arr (strict)"("HorizScroll"=w494, "Number of Columns"=w497, "Index Values"=u32[] [0]) -> ()  [unwired: 2 in, 2 out]
      }
      frame "EnableControls" {
        n234 = property class="VI"() -> ("Panel"=w504:refnum<vi>)  [unwired: 2 in, 2 out]
        n235 = property class="Pnl"(reference=w504) -> ("Controls[]"=w503:refnum<vi>[])  [unwired: 1 in, 2 out]
        n236 = property class="Pnl"(reference=w504) -> ("Decos[]"=w505:refnum<vi>[])  [unwired: 1 in, 2 out]
        n237 = for {
          tunnel: w505 -> [w509] mode=indexing
          tunnel: TRUE -> [w508]
          n238 = property class="Decor"(reference=w509, "Visible"=w508) -> ()  [unwired: 1 in, 2 out]
        }
        n239 = for {
          tunnel: w503 -> [w512] mode=indexing
          tunnel: T6."Enabled" ("Disabled") -> [w511]
          tunnel: [w510] -> _
          n240 = property class="Ctl"(reference=w512, "DisabledEnum"=w511) -> (error out=w510:errorcluster)  [unwired: 1 in, 1 out]
        }
      }
      frame "DisableControls" {
        n241 = property class="VI"() -> ("Panel"=w516:refnum<vi>)  [unwired: 2 in, 2 out]
        n242 = property class="Pnl"(reference=w516) -> ("Controls[]"=w515:refnum<vi>[])  [unwired: 1 in, 2 out]
        n243 = property class="Pnl"(reference=w516) -> ("Decos[]"=w517:refnum<vi>[])  [unwired: 1 in, 2 out]
        n244 = for {
          tunnel: w517 -> [w521] mode=indexing
          tunnel: FALSE -> [w520]
          n245 = property class="Decor"(reference=w521, "Visible"=w520) -> ()  [unwired: 1 in, 2 out]
        }
        n246 = for {
          tunnel: w515 -> [w524] mode=indexing
          tunnel: T6."Disabled and Grayed Out" ("Disabled") -> [w523]
          tunnel: [w522] -> _
          n247 = property class="Ctl"(reference=w524, "DisabledEnum"=w523) -> (error out=w522:errorcluster)  [unwired: 1 in, 1 out]
        }
      }
      frame "Error" {
        w525 = T5[] [enum."Exit"] items=["Idle", "Init", "SetInpChanEnable", "SetInpChanOffset", "SetInpChanTrg", "SetSyncDivider", "SetSyncTrg", "SetSyncOffset", "SetBinning", "SetHistoOffset", "SetHistoLen", "SetStopOvl", "SetBitShift", "SetHistoAcqTime", "GetRates", "GetAllRates", "StartMeas", "StopMeas", "AbortMeas", "GetResolution", "GetHistos", "GetAllHistos", "ReadFiFo", "WriteStatus", "Resize", "EnableControls", "DisableControls", "Error", "Exit"]
        w528 = T10 1 items=["no dialog", "OK message", "continue or stop message", "OK message + warnings", "continue/stop + warnings"] ("type of dialog (OK msg:1)")
        # "Error case: If an error occures the user is informed and the programm terminates. Add your own code to handle error events (e.g. exception lists, etc.)"
        n248 = call <vilib>:"Simple Error Handler.vi"("type of dialog (OK msg:1)"=w528, "error in (no error)"=w527) -> ()  [unwired: 3 in, 5 out]
      }
      frame "Exit" {
        n249 = Unbundle By Name(w532) -> ("DevIdx"=w531:i32)
        n250 = call "MH_CloseDevice.vi"("devidx"=w531) -> ("error out"=w530:errorcluster)  [unwired: 9 in, 1 out]
      }
    }
    n251 = call "MH_EnQError.vi"("error in (no error)"=w8, "Cmds_in"=w6) -> ("error out"=w7:errorcluster, "Cmds_out"=w5:T5[])  [unwired: 8 in]
  }
